vi "to string.vi"(8 "error in":errorcluster, 11 "TEC configuration in":refnum<class "TEC configuration.lvclass">) -> (0 "error out":errorcluster, 1 "data":string, 2 "version":string, 3 "TEC configuration out":refnum<class "TEC configuration.lvclass">)   [LabVIEW 2013, in "TEC configuration.lvclass"]
doc: "Provides an interface for saving a module configuration to a file or other serialized data source. It is recommended that all children of this class store data in two sets--data required for its own initialization, and any data required for parent initialization--and that each implementation uses the <b>Call Parent Method</b> primitive to serialize parent information."
uses:
  TEC configuration.lvclass
  <vilib>/NI/Tag Bus Module Framework/module configuration/TBM module configuration.lvclass
  TEC configuration.lvclass/TEC configuration.ctl
  <vilib>/NI/Configuration Framework/serializable configuration/NISE_CEF_serializable configuration.lvclass
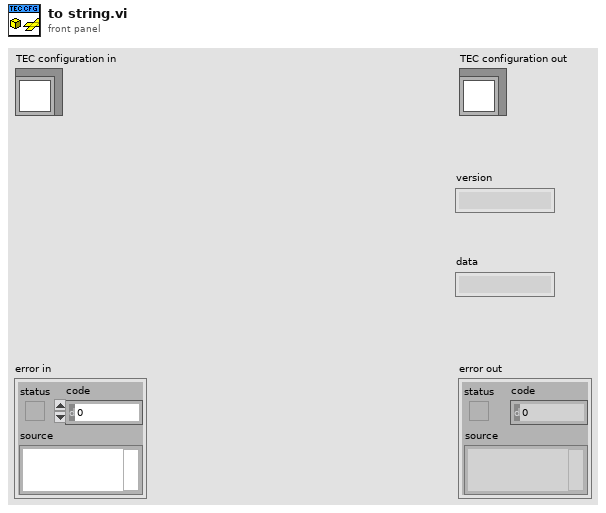
[diagram p1: front panel]
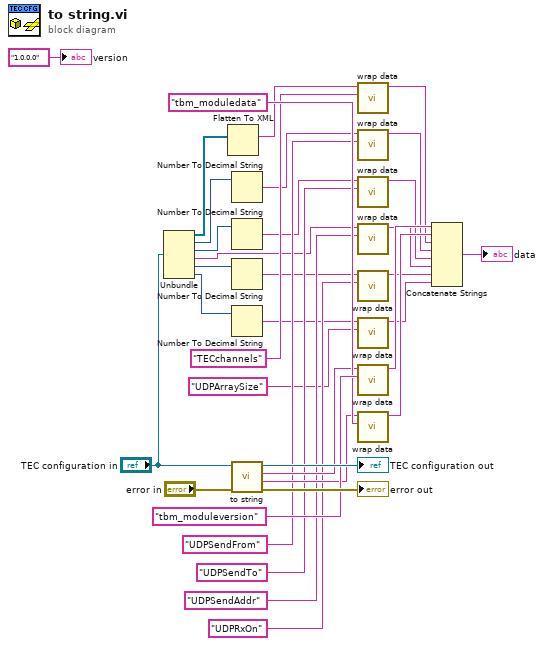
[diagram p0: block diagram]
diagram:
  n1 = Unbundle("TEC configuration in") -> (w24:refnum<class "TBM channel.lvclass">[], w11:u16, w8:u16, w7:string, w6:u16, w1:u16)
  n2 = Flatten To XML(anything=w24) -> (xml string=w23:string)
  n3 = Number To Decimal String(number=w11) -> (decimal integer string=w10:string)  [unwired: 1 in]
  n4 = Number To Decimal String(number=w8) -> (decimal integer string=w9:string)  [unwired: 1 in]
  n5 = Number To Decimal String(number=w6) -> (decimal integer string=w5:string)  [unwired: 1 in]
  n6 = Number To Decimal String(number=w1) -> (decimal integer string=w4:string)  [unwired: 1 in]
  n7 = call-parent "to string.vi"("error in"="error in", "module configuration in"="TEC configuration in") -> ("error out"=→"error out":errorcluster, "data"=w27:string, "version"=w28:string, "module configuration out"=→"TEC configuration out":refnum<class "TEC configuration.lvclass">)  [unwired: 6 in]
  n8 = call <vilib>:"wrap data.vi"("identifier"="TECchannels" ("additional identifier"), "data to wrap"=w23) -> ("wrapped data"=w22:string)  [unwired: 9 in]
  n9 = call <vilib>:"wrap data.vi"("identifier"="UDPSendFrom" ("additional identifier"), "data to wrap"=w10) -> ("wrapped data"=w15:string)  [unwired: 9 in]
  n10 = call <vilib>:"wrap data.vi"("identifier"="UDPSendTo" ("additional identifier"), "data to wrap"=w9) -> ("wrapped data"=w14:string)  [unwired: 9 in]
  n11 = call <vilib>:"wrap data.vi"("identifier"="UDPSendAddr" ("additional identifier"), "data to wrap"=w7) -> ("wrapped data"=w13:string)  [unwired: 9 in]
  n12 = call <vilib>:"wrap data.vi"("identifier"="UDPRxOn" ("additional identifier"), "data to wrap"=w5) -> ("wrapped data"=w12:string)  [unwired: 9 in]
  n13 = call <vilib>:"wrap data.vi"("identifier"="UDPArraySize" ("additional identifier"), "data to wrap"=w4) -> ("wrapped data"=w2:string)  [unwired: 9 in]
  n14 = call <vilib>:"wrap data.vi"("identifier"="tbm_moduleversion" ("additional identifier"), "data to wrap"=w28) -> ("wrapped data"=w30:string)  [unwired: 9 in]
  n15 = call <vilib>:"wrap data.vi"("identifier"="tbm_moduledata" ("additional identifier"), "data to wrap"=w27) -> ("wrapped data"=w29:string)  [unwired: 9 in]
  n16 = Concatenate Strings(w30, w29, w22, w15, w14, w13, w12, w2) -> (→"data":string)
  "version" <- "1.0.0.0" ("current version")
